vi "PH_ImageOperator.Lev-Mar xx.vi"(4 "No Offset?":bool, 5 "Standard Deviation":dbl[](array[numeric]) format="%0.2f", 6 "Order of GAUSSian function":i32, 7 "error":i32, 8 "Coefficients":dbl[](array[numeric]) format="%0.2f", 9 "Y":dbl[](array[numeric]) format="%0.2f", 10 "X":dbl[](array[numeric]) format="%0.2f") -> (1 "chiSqr":dbl format="%0.2f")   [LabVIEW 2014, in "PH_ImageOperator.lvlib"]
uses:
  PH_ImageOperator.lvlib
panel:
  # "Lev-Mar\nXX"
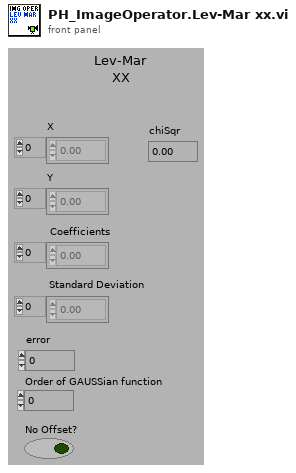
[diagram p1: front panel]
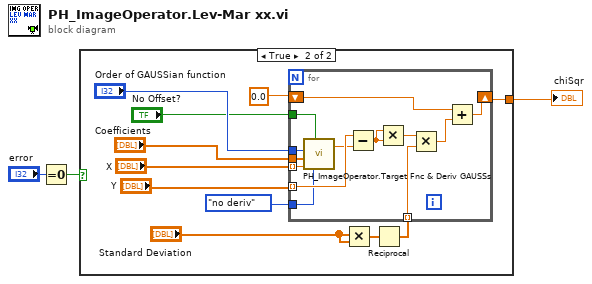
[diagram p0: block diagram]
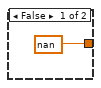
[diagram p2: hidden frame]
diagram:
  n1 = Equal To 0?(x="error") -> (x = 0?=w2:bool)
  n2 = case shown="True" w2 {
    tunnel: [nan w14] -> w1
    frame False {
    }
    frame True {
      n3 = Multiply(x="Standard Deviation", y="Standard Deviation") -> (x*y=w9:dbl[])
      n4 = Reciprocal(x=w9) -> (1/x=w8:dbl[])
      n5 = for {
        shift-right: [w27] -> w14
        shift-left: 0.0 -> [w28]
        tunnel: "Y" -> [w26] mode=indexing
        tunnel: "Coefficients" -> [w24]
        tunnel: "X" -> [w23] mode=indexing
        tunnel: w8 -> [w19] mode=indexing
        tunnel: "Order of GAUSSian function" -> [w18]
        tunnel: enum16{"no deriv", "deriv"}."no deriv" -> [w17]
        tunnel: "No Offset?" -> [w16]
        n6 = call "PH_ImageOperator.Target Fnc & Deriv GAUSSs.vi"("Flag"=w17, "Order of GAUSSian function"=w18, "Coefficients"=w24, "X"=w23, "No Offset?"=w16) -> ("Y"=w22:dbl)  [unwired: 1 out]
        n7 = Subtract(x=w26, y=w22) -> (x-y=w25:dbl)
        n8 = Multiply(x=w25, y=w25) -> (x*y=w20:dbl)
        n9 = Multiply(x=w20, y=w19) -> (x*y=w21:dbl)
        n10 = Add(x=w28, y=w21) -> (x+y=w27:dbl)
      }
    }
  }
  "chiSqr" <- w1
